vi "Velocity (Reframed) Get.vi"(8 "error in (no error)":errorcluster, 10 "Frame Properties (m)":T1) -> (0 "error out":errorcluster, 2 "Reframed Velocity (m/s)":T2 {"vz (m/s)" format="%.1f"; "vy (m/s)" format="%.1p"; "vx (m/s)" format="%.1p"})   [LabVIEW 2021, in "Haptic Prog Interface.lvlib"]
doc: "Returns the horizontal xy-velocities of the haptic pen in nm/s, and the vertical z-position in mm/s. The horizontal velocity depends on the frame origin and frame size.\n\n<b>Velocity:</b> Returns a cluster of the x (nm/s), y (nm/s), and z (mm/s) velocities of the pen."
uses:
  Haptic Prog Interface.lvlib
  Haptic-Programming-Interface/src/x64/Debug/Haptic Programming Interface.dll
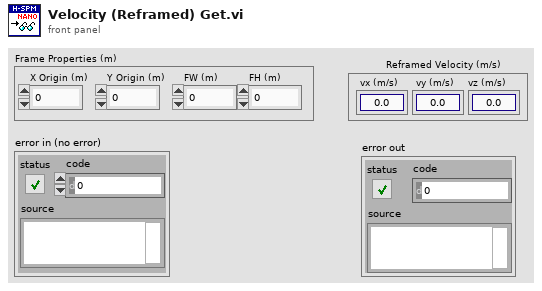
[diagram p1: front panel]
types:
  T1 = cluster{"X Origin (m)":dbl, "Y Origin (m)":dbl, "FW (m)":dbl, "FH (m)":dbl}
  T2 = cluster{"vx (m/s)":dbl, "vy (m/s)":dbl, "vz (m/s)":dbl}
  T3 = cluster{"vx (m/s)":dbl, "vy (m/s)":dbl, "vz (mm/s)":dbl}
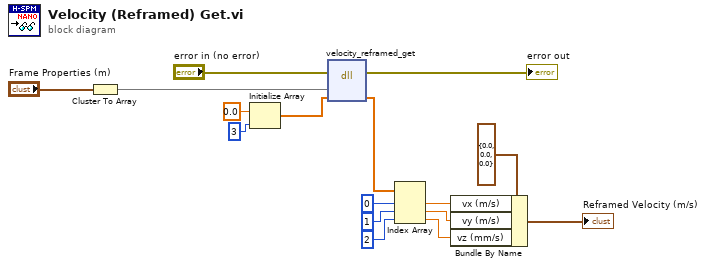
[diagram p0: block diagram]
diagram:
  n1 = Cluster To Array(cluster="Frame Properties (m)") -> (array=w7:dbl[])
  n2 = Initialize Array(0.0 ("element"), 3 ("dimension size")) -> (w2:dbl[])
  n3 = dll-call lib="C:/Users/freem/Documents/GitHub/Haptic-Programming-Interface/src/x64/Debug/Haptic Programming Interface.dll" fn="velocity_reframed_get"(error in="error in (no error)", "frame_properties"=w7, "output"=w2) -> (error out=→"error out":errorcluster, "output"=w15:dbl[])  [unwired: 4 in, 1 out]
  n4 = Index Array(array=w15, index #1=0 ("index"), index #2=1 ("index"), index #3=2 ("index")) -> (element #1=w10:dbl, element #2=w9:dbl, element #3=w11:dbl)
  n5 = Bundle By Name(cluster=T3 {"vx (m/s)"=0.0, "vy (m/s)"=0.0, "vz (mm/s)"=0.0} ("Velocity (Reframed)"), "vx (m/s)"=w10, "vy (m/s)"=w9, "vz (mm/s)"=w11) -> (→"Reframed Velocity (m/s)":T3)
